vi "User Event Abort.vi"(8 "Error In":errorcluster, 10 "User Event States":T1) -> (0 "Error Out":errorcluster, 2 "User Event":refnum<user-event>)   [LabVIEW 2015]
doc: "VI used to create, get or destroy or user event for aborting application."
uses:
  Controls/User Events States.ctl
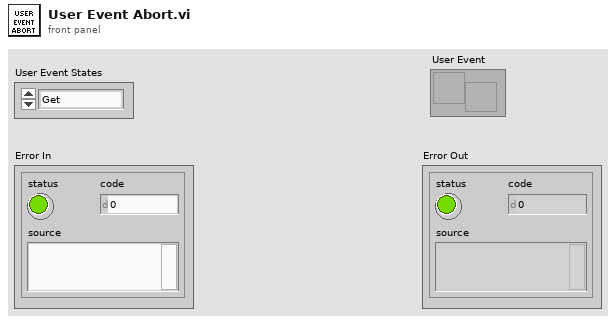
[diagram p1: front panel]
types:
  T1 = typedef "User Events States.ctl" = enum16{"Get", "Create", "Destroy"}
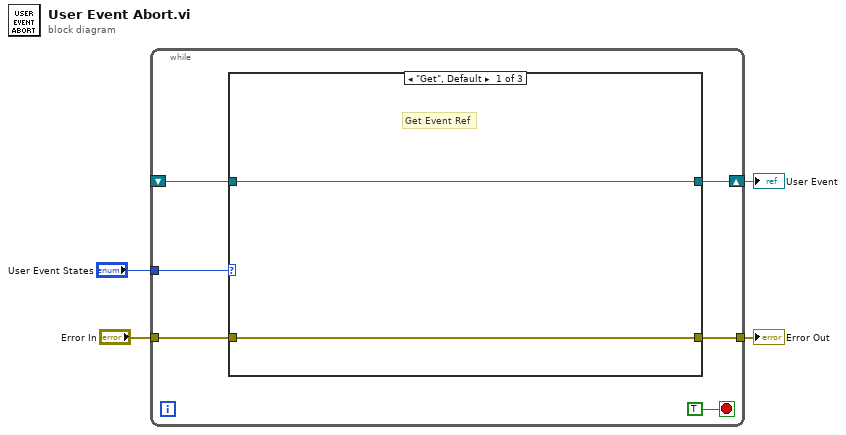
[diagram p0: block diagram]
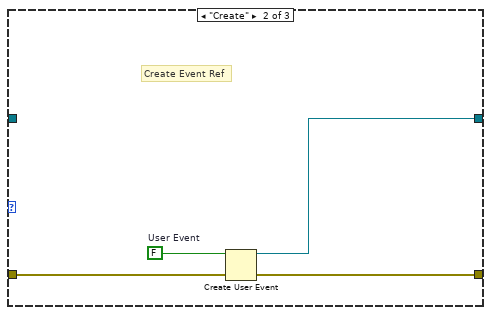
[diagram p2: hidden frame]
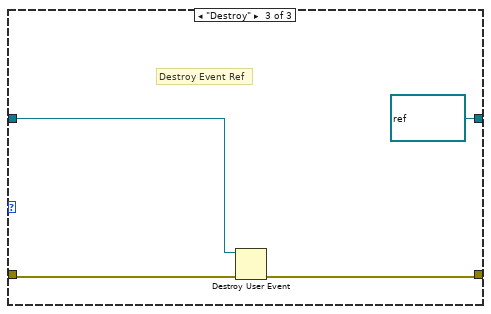
[diagram p3: hidden frame]
diagram:
  n1 = while {
    tunnel: "User Event States" -> [w10]
    tunnel: "Error In" -> [w9]
    tunnel: [w8] -> w2
    shift-right: [w7] -> w1
    shift-left: _ -> [w6]
    stop <- TRUE stop-if-true
    n2 = case shown="\"Get\", Default" w10 {
      tunnel: w9 -> [w11 w16 w20]
      tunnel: [w11 w14 w19] -> w8
      tunnel: [w12 w13 refnum<user-event> refnum ("User Event")] -> w7
      tunnel: w6 -> [w12 _ w18]
      frame "Get", Default {
        # "Get Event Ref"
      }
      frame "Create" {
        w15 = FALSE  # User Event
        # "Create Event Ref"
        n3 = Create User Event(user event datatype=w15, error in=w16) -> (user event=w13:refnum<user-event>, error out=w14:errorcluster)
      }
      frame "Destroy" {
        # "Destroy Event Ref"
        n4 = Destroy User Event(user event=w18, error in=w20) -> (error out=w19:errorcluster)
      }
    }
  }
  "Error Out" <- w2
  "User Event" <- w1
